vi "Get Active String Functions.vi"(0 "String Functions in":refnum<class "String Functions.lvclass">, 11 "error in (no error)":errorcluster) -> (4 "String Functions out":refnum<class "String Functions.lvclass">, 6 "Function List":T1, 15 "error out":errorcluster)   [LabVIEW 2016, in "String Functions.lvclass"]
uses:
  String Functions.lvclass
  E:/Repository/LabVIEW Script Language/source code/LSL components/functions/functionsbase/functionbase.lvclass
  Function List.ctl
  functionsbase/functionbase.lvclass
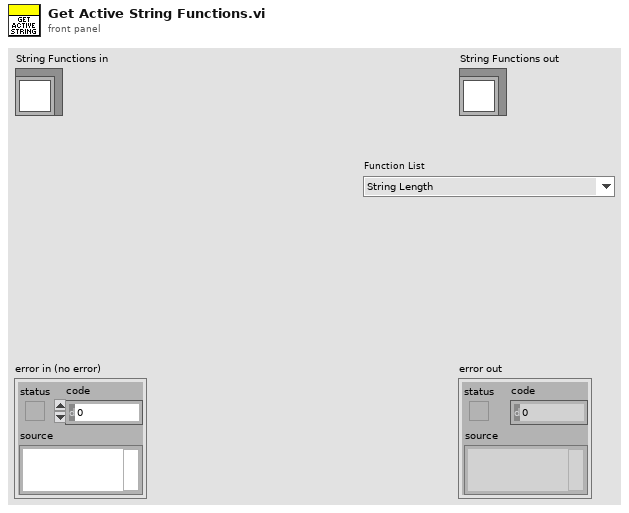
[diagram p1: front panel]
types:
  T1 = typedef "String Functions.lvclass/Function List.ctl" = enum16{"String Length", "Concatenate String", "String Subset", "Replace Substring", "To Upper Case", "To Lower Case", "Convert to String", "String to Number", "Random String", "String Reverse"}
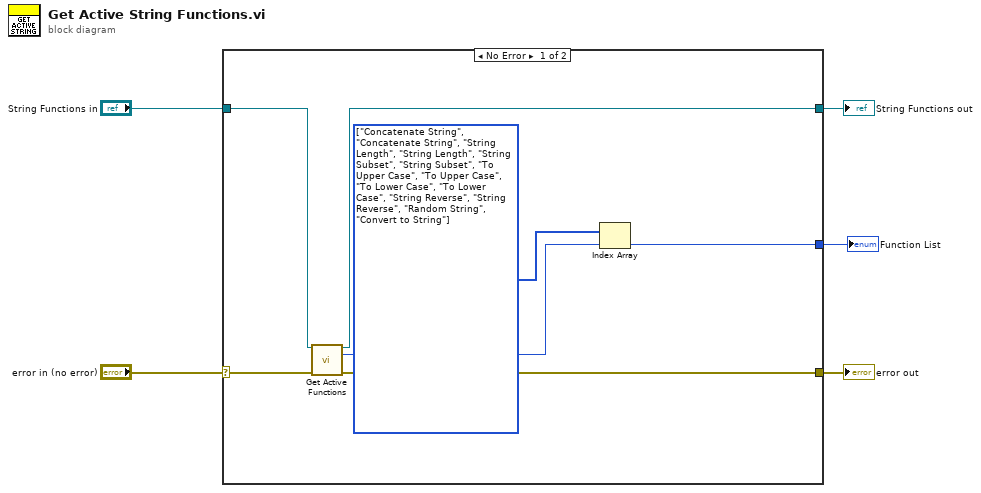
[diagram p0: block diagram]
diagram:
  n1 = case shown="No Error" "error in (no error)" {
    selector: "error in (no error)" -> [w12 w14]
    tunnel: [w11 w14] -> w4
    tunnel: [w9 w13] -> w2
    tunnel: "String Functions in" -> [w10 w13]
    tunnel: [w6 _] -> w1
    frame No Error {
      w8 = T1[] [enum."Concatenate String", enum."Concatenate String", enum."String Length", enum."String Length", enum."String Subset", enum."String Subset", enum."To Upper Case", enum."To Upper Case", enum."To Lower Case", enum."To Lower Case", enum."String Reverse", enum."String Reverse", enum."Random String", enum."Convert to String"] items=["String Length", "Concatenate String", "String Subset", "Replace Substring", "To Upper Case", "To Lower Case", "Convert to String", "String to Number", "Random String", "String Reverse"]
      n2 = call "Get Active Functions.vi"("functionbase in"=w10, "error in (no error)"=w12) -> ("functionbase out"=w9:refnum<class "String Functions.lvclass">, "Syntax Index"=w7:i32, "error out"=w11:errorcluster)  [unwired: 11 in]
      n3 = Index Array(array=w8, index=w7) -> (element=w6:T1)
    }
    frame Error {
    }
  }
  "error out" <- w4
  "String Functions out" <- w2
  "Function List" <- w1
